vi "Sub-CDC_Data_Cluster_Buffer.vi"(7 "Mode":enum16{"Init", "Add", "Add Load", "Out"}(ring), 10 "Input Load":dbl[](array[numeric]), 11 "Input CL":T2) -> (3 "Output CL":T1)   [LabVIEW 2015]
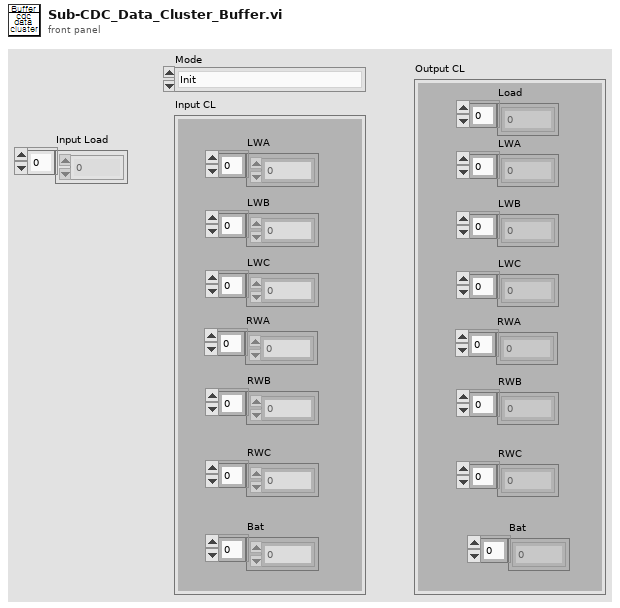
[diagram p1: front panel]
types:
  T1 = cluster{"Load":dbl[], "LWA":dbl[], "LWB":dbl[], "LWC":dbl[], "RWA":dbl[], "RWB":dbl[], "RWC":dbl[], "Bat":u16[]}
  T2 = cluster{"LWA":dbl[], "LWB":dbl[], "LWC":dbl[], "RWA":dbl[], "RWB":dbl[], "RWC":dbl[], "Bat":u16[]}
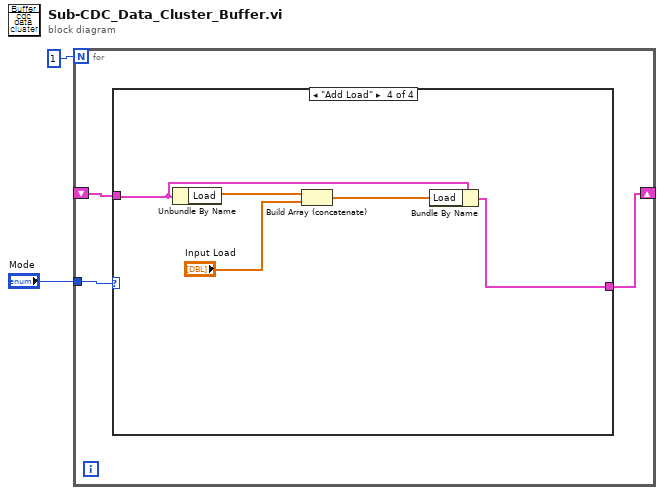
[diagram p0: block diagram]
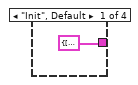
[diagram p2: hidden frame]
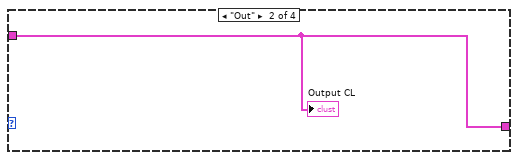
[diagram p3: hidden frame]
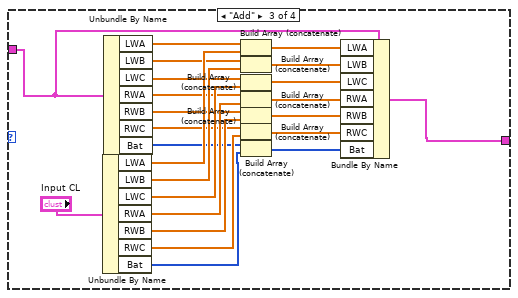
[diagram p4: hidden frame]
diagram:
  n1 = for {
    N: 1 -> [_]
    tunnel: "Mode" -> [w5]
    shift-right: [w4] -> _
    shift-left: _ -> [w3]
    n2 = case shown="\"Add Load\"" w5 {
      tunnel: [T1 {"Load"=[], "LWA"=[], "LWB"=[], "LWC"=[], "RWA"=[], "RWB"=[], "RWC"=[], "Bat"=[]} ("Output CL") w7 w12 w32] -> w4
      tunnel: w3 -> [_ w7 w8 w33]
      frame "Init", Default {
      }
      frame "Out" {
        "Output CL" <- w7
      }
      frame "Add" {
        n3 = Unbundle By Name("Input CL") -> ("LWA"=w29:dbl[], "LWB"=w27:dbl[], "LWC"=w25:dbl[], "RWA"=w23:dbl[], "RWB"=w21:dbl[], "RWC"=w19:dbl[], "Bat"=w10:u16[])
        n4 = Unbundle By Name(w8) -> ("LWA"=w30:dbl[], "LWB"=w28:dbl[], "LWC"=w26:dbl[], "RWA"=w24:dbl[], "RWB"=w22:dbl[], "RWC"=w20:dbl[], "Bat"=w11:u16[])
        n5 = Build Array (concatenate)(w30, w29) -> (w18:dbl[])
        n6 = Build Array (concatenate)(w28, w27) -> (w17:dbl[])
        n7 = Build Array (concatenate)(w26, w25) -> (w16:dbl[])
        n8 = Build Array (concatenate)(w24, w23) -> (w15:dbl[])
        n9 = Build Array (concatenate)(w22, w21) -> (w14:dbl[])
        n10 = Build Array (concatenate)(w20, w19) -> (w13:dbl[])
        n11 = Build Array (concatenate)(w11, w10) -> (w9:u16[])
        n12 = Bundle By Name(cluster=w8, "LWA"=w18, "LWB"=w17, "LWC"=w16, "RWA"=w15, "RWB"=w14, "RWC"=w13, "Bat"=w9) -> (w12:T1)
      }
      frame "Add Load" {
        n13 = Unbundle By Name(w33) -> ("Load"=w36:dbl[])
        n14 = Build Array (concatenate)(w36, "Input Load") -> (w34:dbl[])
        n15 = Bundle By Name(cluster=w33, "Load"=w34) -> (w32:T1)
      }
    }
  }
